vi "MoveAbsSingle.vi"(5 "position":dbl, 7 "speed":dbl min=0.0, 8 "error in (no error)":errorcluster, 9 "taskId":i32(ring) items=["TLibrary", "T01", "T02", "T03", "T04", "T05", "T06", "T07", "T08", "T09", "T10", "T11", "T12", "T13", "T14", "T15", "T16", "T17", "T18", "T19", "T20", "T21", "T22", "T23", "T24", "T25", "T26", "T27", "T28", "T29", "T30", "T31"], 10 "axis name":string, 11 "controller in":refnum<k24>) -> (0 "error out":errorcluster, 3 "controller out":refnum<k24>)   [LabVIEW 2010]
uses:
  c:/aerotech/controller/stable/A3200/pc/labview/2010/bin/Aerotech.A3200.dll
  bin/Aerotech.A3200.dll
  c:/aerotech/controller/stable/A3200/pc/labview/2010/bin/Aerotech.A3200.LabVIEW.dll
  bin/Aerotech.A3200.LabVIEW.dll
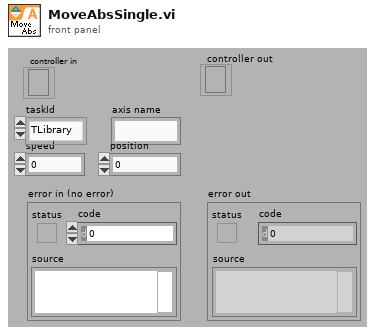
[diagram p1: front panel]
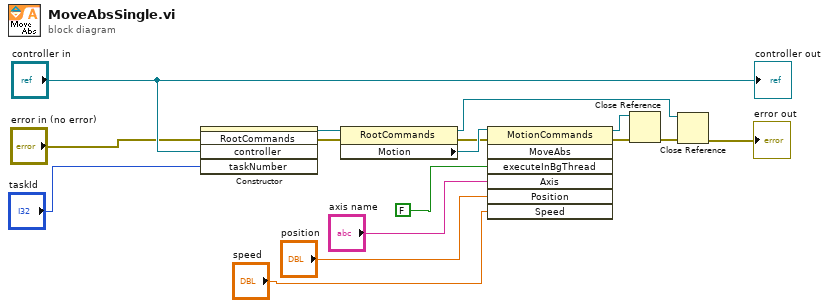
[diagram p0: block diagram]
diagram:
  n1 = constructor class="RootCommands"(error in="error in (no error)", "controller"="controller in", "taskNumber"="taskId") -> (reference out=w9:refnum<k24>, error out=w8:errorcluster)  [unwired: 2 in, 3 out]
  n2 = property class="RootCommands"(reference=w9, error in=w8) -> (reference out=w4:refnum<k24>, error out=w10:errorcluster, "Motion"=w11:refnum<k24>)
  n3 = invoke class="MotionCommands" method="MoveAbs"(reference=w11, error in=w10, "executeInBgThread"=FALSE, "Axis"="axis name", "Position"="position", "Speed"="speed") -> (reference out=w6:refnum<k24>, error out=w7:errorcluster)  [unwired: 1 in, 5 out]
  n4 = Close Reference(reference=w6, error in (no error)=w7) -> (error out=w5:errorcluster)
  n5 = Close Reference(reference=w4, error in (no error)=w5) -> (error out=→"error out":errorcluster)
  "controller out" <- "controller in"
